vi "Stereo Wav File Test.vi"() -> ()   [LabVIEW 2015]
uses:
  Controls/Waveform XCtl/Waveform Enum.ctl
  Controls/Level XCtl/Level Modes.ctl
  Top Level VIs/Stimulus-Initialize (full array).vi
  Controls/Stimulus Channel (Full)/Stimulus Channel (Full).xctl
panel:
  out "Waveform Graph":dbl[][](graph)
  in  "Waveform.File.Filename":path
  in  "Dummy":T22(xcontrol)
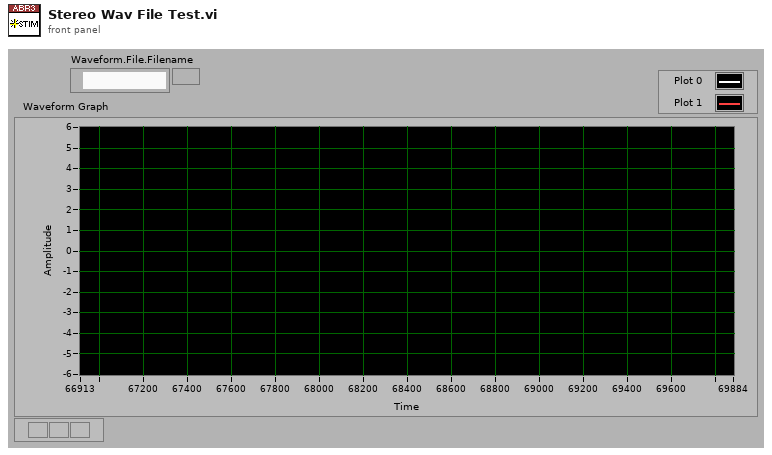
[diagram p1: front panel]
types:
  T1 = typedef "Waveform XCtl.xctl/Waveform Data.ctl" = cluster{"Type":T2, "Tone":T3, "Pulse Train":T4, "Noise":T7, "File":T8, "FMSweep":T9, "Chirp Train":T10, "Complex Tone":cluster{"Params":T12, "Data":T14}}
  T2 = typedef "Waveform Enum.ctl" = enum16{"OFF", "Tone", "Noise", "Pulse Train", "File", "FM Sweep", "Chirp Train", "Complex Tone"}
  T3 = typedef "Tone Params.ctl" = cluster{"Frequency (kHz)":dbl, "Last Freq":dbl, "Last Phase":dbl}
  T4 = typedef "Pulse Train Params.ctl" = cluster{"Pulse width (us)":dbl, "Pulse rate (Hz)":dbl, "Gap (ms)":dbl, "Polarity":T5, "PT State":T6, "Asynch":bool}
  T5 = typedef "Pulse Polarity.ctl" = enum16{"POS", "NEG", "POS-NEG", "NEG-POS"}
  T6 = typedef "PT-Continuous State.ctl" = cluster{"Template":dbl[], "Nperiod":i32, "Index":i32, "Pulse Rate (Hz)":dbl, "Phase (cycles)":dbl, "Noff":i32}
  T7 = typedef "Noise Params.ctl" = cluster{"InvFilt":bool, "Noise":dbl[], "CurPt":i32, "Aweight":bool}
  T8 = typedef "StimFile-Params.ctl" = cluster{"Filename":path, "Signal":dbl[], "Channel":i32}
  T9 = typedef "FM Sweep Params.ctl" = cluster{"Rate (oct/s)":dbl, "Fmin (Hz)":dbl, "Fmax (Hz)":dbl, "Ramp (ms)":dbl, "Linear":bool}
  T10 = typedef "Chirp Train.ctl" = cluster{"Params":T11, "Data":cluster{"WF":dbl[]}}
  T11 = typedef "Chirp Train Params.ctl" = cluster{"Fmin (kHz)":dbl, "Fmax (kHz)":dbl, "Compensate":bool, "Duration (ms)":dbl}
  T12 = typedef "CT-Params.ctl" = cluster{"F0 (Hz)":dbl, "Band":cluster{"Flow (Hz)":dbl, "Fhigh (Hz)":dbl}, "Phase":T13, "Min F0 (Hz)":dbl, "Max F0 (Hz)":dbl, "ContinRandPhase":bool, "Max peak factor":dbl, "Max mod depth":dbl}
  T13 = typedef "CT-Phase Enum.ctl" = enum16{"Cosine", "Random", "Alternating"}
  T14 = typedef "CT-Runtime Data.ctl" = cluster{"Ncomp":i32, "MinHarm":i32, "Phase":dbl[], "Amplitude":dbl[], "Npts/frame":i32, "Last F0":dbl, "Fmin":dbl, "Fmax":dbl, "Lslope":dbl, "randphase":bool}
  T15 = typedef "Advanced Filter XCtl.xctl/Filter Data.ctl" = cluster{"Type":enum16{"Lowpass", "Highpass", "Bandpass", "Bandstop", "OFF"}, "CF (kHz)":dbl, "BW (kHz)":dbl, "Cascade":bool, "Quadrature":bool, "Scale Factor":dbl, "Stages":cluster{"IIR Filter":cluster{"filter structure":enum32{"IIR 2nd Order", "IIR 4th Order"}, "Reverse Coefficients":dbl[], "Forward Coefficients":dbl[]}, "State":dbl[]}[], "Class":enum16{"Elliptic", "Butterworth"}, "Order":i32, "BWUnits":T16}
  T16 = typedef "Filter-Bandwidth Units.ctl" = enum16{"Linear", "Octaves"}
  T17 = typedef "Burst Control.xctl/Burst Data.ctl" = cluster{"Active":bool, "Delay (ms)":dbl, "Duration (ms)":dbl, "Ramp (ms)":dbl, "Rate (Hz)":dbl, "Trepeat (ms)":dbl, "Repeat":bool}
  T18 = typedef "Level XCtl.xctl/Level Data.ctl" = cluster{"Level":dbl, "Units":T19, "Max":dbl, "Multiplier":dbl, "Cal File":path, "Cal":cluster{"Freq (Hz)":dbl[], "Mag (dB SPL)":dbl[], "Phase (deg)":dbl[]}}
  T19 = typedef "Level Units.ctl" = enum16{"dB atten", "dB SPL", "dB re 1 Vrms", "dB V/Hz½", "mW", "dB SL"}
  T20 = typedef "Advanced Stimulus Options.xctl/Advanced Stimulus Options.ctl" = cluster{"Rep Mask":string, "AltPol":bool, "Var":string, "Expr":string}
  T21 = typedef "SAM Params.ctl" = cluster{"Active":bool, "Frequency (Hz)":dbl, "Depth":dbl, "Init Phase (cycles)":dbl, "phase (degrees)":dbl, "Asynch":bool}
  T22 = cluster{"Waveform":T1, "Filter":T15, "Burst":T17, "Level":T18, "Name":string, "Advanced":T20, "SAM":T21}
  T23 = enum16{"Lowpass", "Highpass", "Bandpass", "Bandstop", "OFF"}
  T24 = typedef "Level Modes.ctl" = enum16{"dB atten", "dB SPL", "dB re 1 Vrms", "dB V/Hz½", "mW"}
  T25 = cluster{"Waveform":T1, "Filter":T15, "Burst":T17, "Level":T18, "Name":string, "Advanced":T20, "SAM":T21}[]
  T26 = typedef "Stimulus Channel (Full).xctl/Full Stimulus Channel Data.ctl" = cluster{"Waveform":T1, "Filter":T15, "Burst":T17, "Level":T18, "Name":string, "Advanced":T20, "SAM":T21}
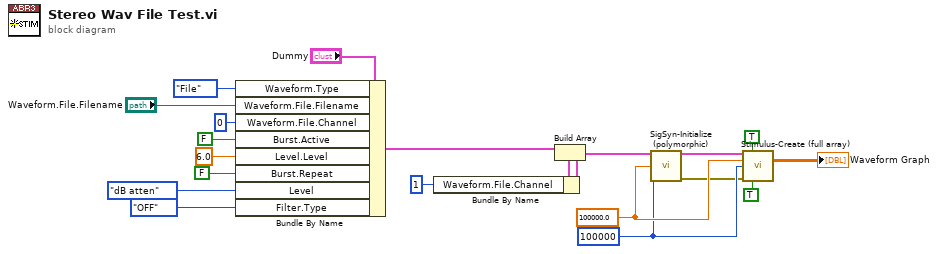
[diagram p0: block diagram]
diagram:
  w3 = 100000 ("Npts")
  w4 = 100000.0 ("Sampling rate (Hz)")
  n1 = Bundle By Name(cluster="Dummy", "Waveform.Type"=Waveform_Enum."File", "Waveform.File.Filename"="Waveform.File.Filename", "Waveform.File.Channel"=0, "Burst.Active"=FALSE, "Level.Level"=6.0, "Burst.Repeat"=FALSE, "Level"=Level_Modes."dB atten" ("Level.Mode"), "Filter.Type"=T23."OFF") -> (w17:T22)
  n2 = Bundle By Name(cluster=w17, "Waveform.File.Channel"=1) -> (w14:T22)
  n3 = Build Array(w17, w14) -> (w8:T25)
  n4 = call-poly "SigSyn-Initialize (polymorphic).vi"("StimChans"=w8, "Sampling rate (Hz)"=w4, "Npts"=w3) -> ("StimChans Out"=w5:T26[], "error out"=w2:errorcluster)  [unwired: 10 in, 1 out]
  n5 = call "Stimulus-Create (full array).vi"("StimChan"=w5, "Apply multipliers? (F)"=TRUE, "Sampling Rate (Hz)"=w4, "Npts"=w3, "error in (no error)"=w2, "Zero unused (F)"=TRUE) -> ("Waveform"=→"Waveform Graph":dbl[][])  [unwired: 6 in, 3 out]
